vi "3458A Setup Virtual Channels.vi"(4 "LEVEL trigger":T1 caption="Cluster", 5 "sample period [s] (1 ms)":dbl=0.001 format="%#_6p", 6 "TRIG source (AUTO)":T2, 7 "apperture [s] (1.4 us)":dbl=1.4e-06 format="%#_6p", 8 "error in":errorcluster, 9 "samples count (100)":i32=100, 10 "voltage ranges [Vpk] (empty: use global default)":dbl[](array[numeric]), 11 "digitizer in":T3 {"channels"."Range [Vpk]" min=0.0}) -> (0 "error out":errorcluster, 3 "digitizer out":T3 {"channels"."Range [Vpk]" min=0.0})   [LabVIEW 2018, in "3458A Virtual Digitizer.lvlib"]
doc: "This VI setups all channels of a virtual digitizer to desired modes. If vector of ranges is entered it will override default channel settings from the session. It also setups all related instruments to the needed states (AWG and counter). Call this VI at least once before initiating digitizing!"
uses:
  3458A Virtual Digitizer.lvlib
  3458A Digitizer Session.ctl
  3458A Virtual Channel Config.ctl
  Counter/Counter Session.ctl
  Counter/Counter Type.ctl
  AWG/AWG Session.ctl
  AWG/AWG Type.ctl
  3458A Sync Mode.ctl
  3458A Idn Mode.ctl
  3458A Digitizing Low Levels/Configure/Sampling Mode.ctl
  3458A Digitizing Process Options.ctl
  3458A Data Packet.ctl
  3458A Aux Record Data.ctl
  3458A Digitizing Low Levels/Configure/Level Setup.ctl
  3458A Digitizing Low Levels/Configure/First Sample Trigger.ctl
  3458A Aperture Selection Mode.ctl
  3458A Digitizing Low Levels/Configure/EXT OUT mode.ctl
  <vilib>/Utility/error.llb/Error Cluster From Error Code.vi
  <vilib>/ErrorRing/Error Ring.xnode
  3458A Digitizing Low Levels/3458A Digitizing Low Levels.lvlib
  AWG/AWG.lvlib
  Counter/Counter.lvlib
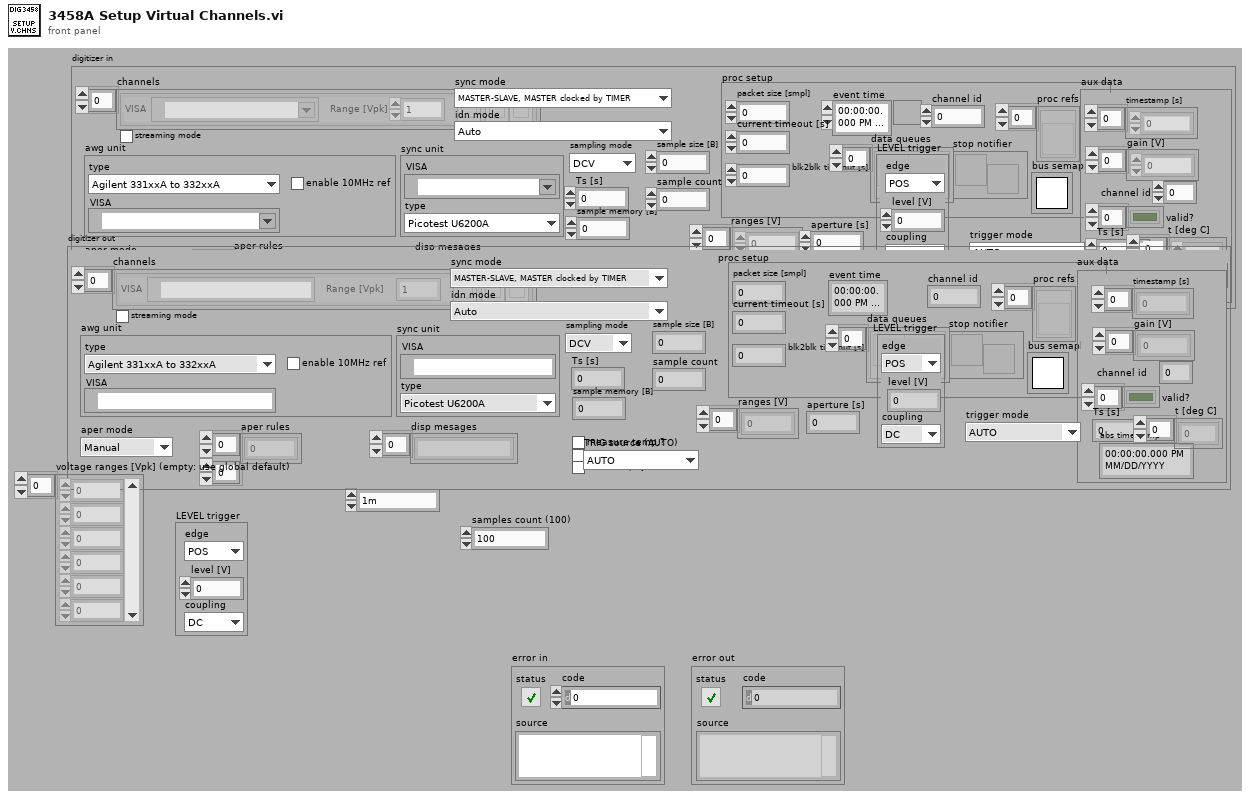
[diagram p1: front panel]
types:
  T1 = typedef "3458A Virtual Digitizer.lvlib/3458A Digitizing Low Levels.lvlib/Level Setup.ctl" = cluster{"edge":enum16{"POS", "NEG"}, "level [V]":dbl, "coupling":enum16{"DC", "AC"}}
  T2 = typedef "3458A Virtual Digitizer.lvlib/3458A Digitizing Low Levels.lvlib/First Sample Trigger.ctl" = enum16{"AUTO", "EXT", "SYN", "SGL", "HOLD", "LEVEL"}
  T3 = typedef "3458A Virtual Digitizer.lvlib/3458A Digitizer Session.ctl" = cluster{"channels":T4[], "sync unit":T5, "awg unit":T7, "sync mode":T9, "streaming mode":bool, "idn mode":T10, "sampling mode":T11, "Ts [s]":dbl, "sample memory [B]":i32, "proc setup":T12, "sample size [B]":i32, "sample count":i32, "aux data":T14, "ranges [V]":dbl[], "aperture [s]":dbl, "LEVEL trigger":T1, "trigger mode":T2, "measure temp.?":bool, "disp mesages":string[], "shared bus?":bool, "disable display?":bool, "aper mode":T15, "aper rules":dbl[][]}
  T4 = typedef "3458A Virtual Digitizer.lvlib/3458A Virtual Channel Config.ctl" = cluster{"VISA":refnum<visa-resource-name>, "Range [Vpk]":dbl, "btn clr":bool, "btn up":bool, "btn down":bool}
  T5 = typedef "Counter.lvlib/Counter Session.ctl" = cluster{"VISA":refnum<visa-resource-name>, "type":T6}
  T6 = typedef "Counter.lvlib/Counter Type.ctl" = enum16{"Picotest U6200A", "dummy"}
  T7 = typedef "AWG.lvlib/AWG Session.ctl" = cluster{"type":T8, "VISA":refnum<visa-resource-name>, "enable 10MHz ref":bool}
  T8 = typedef "AWG.lvlib/AWG Type.ctl" = enum16{"Agilent 331xxA to 332xxA", "Agilent 335xxA to 336xxA", "Tektronix AFG3101C", "dummy"}
  T9 = typedef "3458A Virtual Digitizer.lvlib/3458A Sync Mode.ctl" = enum16{"MASTER-SLAVE, MASTER clocked by TIMER", "MASTER-SLAVE, MASTER clocked by AWG", "ALL clocked by AWG", "MASTER-SLAVE, ALL clocked by TIMER", "ALL clocked by AWG with DFLL"}
  T10 = typedef "3458A Virtual Digitizer.lvlib/3458A Idn Mode.ctl" = enum16{"Auto", "Sequential (chn A, chn B, ...)", "From calibration string"}
  T11 = typedef "3458A Virtual Digitizer.lvlib/3458A Digitizing Low Levels.lvlib/Sampling Mode.ctl" = enum16{"DCV", "DSDC", "DSAC"}
  T12 = typedef "3458A Virtual Digitizer.lvlib/3458A Digitizing Process Options.ctl" = cluster{"channel id":i32, "packet size [smpl]":i32, "current timeout [s]":dbl, "blk2blk timeout [s]":dbl, "event time":timestamp, "stop notifier":refnum<notifier>, "data queues":refnum<queue>[], "proc refs":refnum<vi>[], "bus semaphore":T13}
  T13 = typedef "Semaphore RefNum" = refnum<k1>
  T14 = typedef "3458A Virtual Digitizer.lvlib/3458A Aux Record Data.ctl" = cluster{"channel id":i32, "valid?":bool[], "gain [V]":dbl[], "timestamp [s]":dbl[], "Ts [s]":dbl, "abs timestamp":timestamp, "t [deg C]":dbl[]}
  T15 = typedef "3458A Virtual Digitizer.lvlib/3458A Aperture Selection Mode.ctl" = enum16{"Manual", "Maximum", "Table"}
  T16 = typedef "3458A Virtual Digitizer.lvlib/3458A Digitizing Low Levels.lvlib/EXT OUT mode.ctl" = enum16{"APER", "ICOMP"}
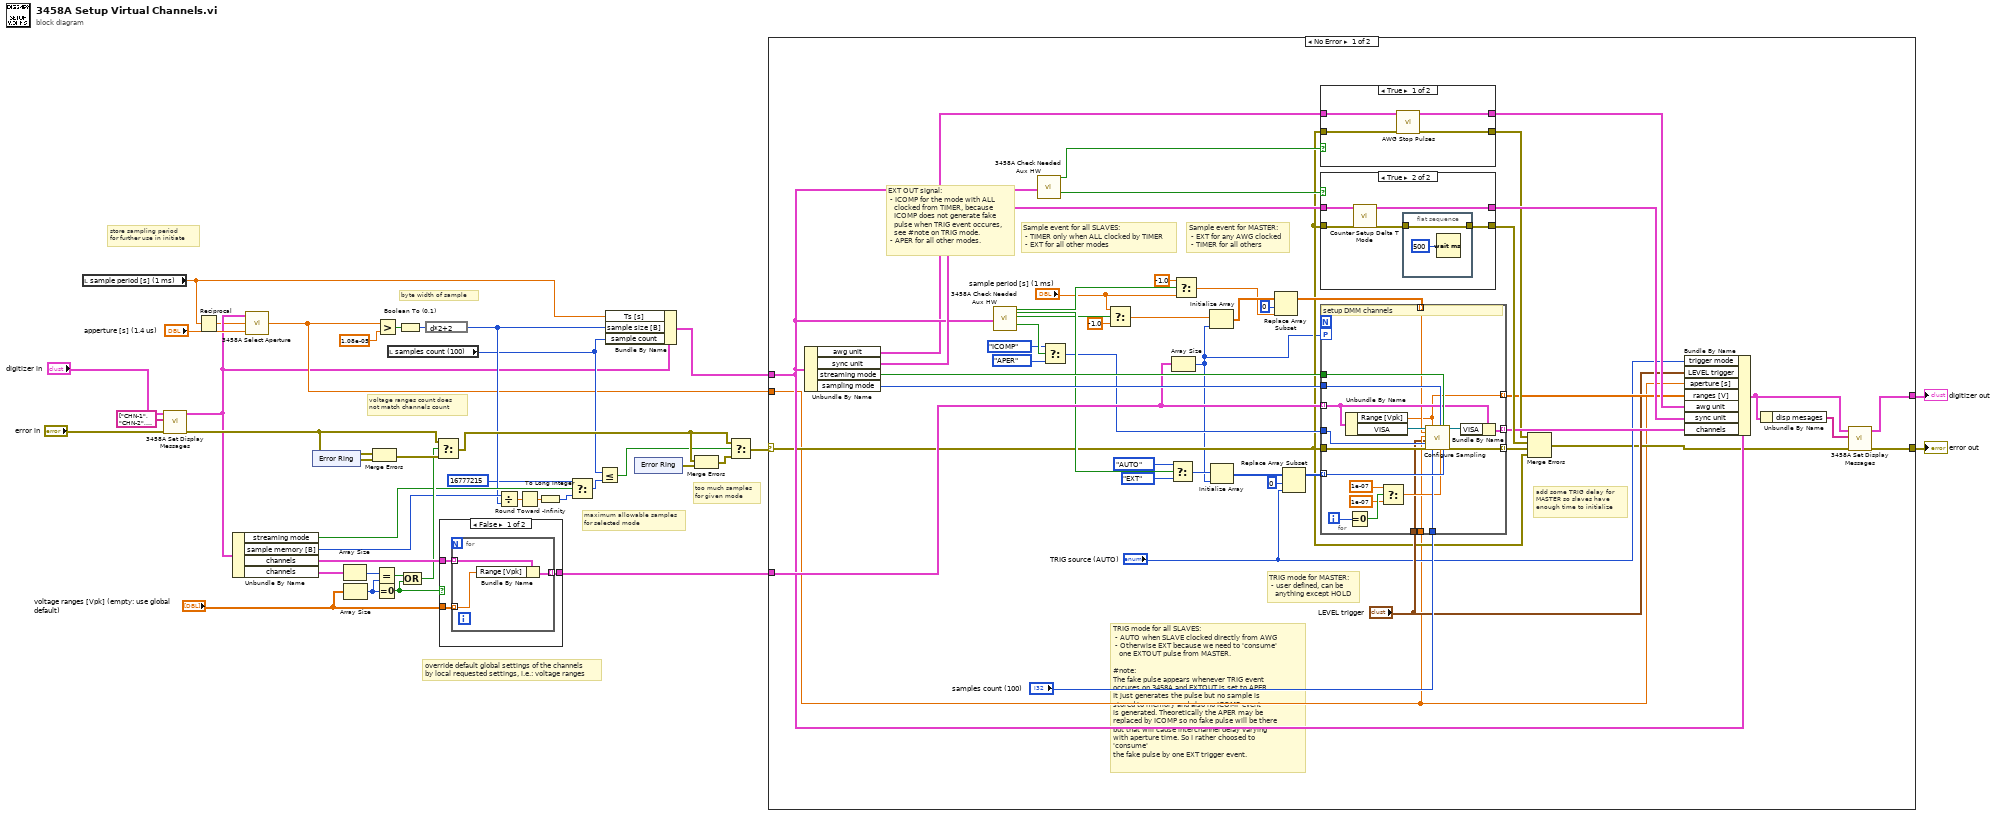
[diagram p0: block diagram]
diagram:
  # "store sampling period\nfor further use in initiate"
  # "voltage ranges count does\nnot match channels count"
  # "maximum allowable samples\nfor selected mode"
  # "byte width of sample"
  # "too much samples\nfor given mode"
  # "override default global settings of the channels\nby local requested settings, i.e.: voltage ranges"
  n1 = local read "sample period [s] (1 ms)"() -> (w2:dbl)
  n2 = call "3458A Set Display Messages.vi"("error in (no error)"="error in", "display strings"=string[] ["CHN-1", "CHN-2", "CHN-3"], "digitizer session in"="digitizer in") -> ("error out"=w8:errorcluster, "digitizer session out"=w3:T3)  [unwired: 7 in]
  n3 = Reciprocal(x=w2) -> (1/x=w1:dbl)
  n4 = Unbundle By Name(w3) -> ("streaming mode"=w21:bool, "sample memory [B]"=w16:i32, "channels"=w37:T4[], "channels"=w38:T4[])
  n5 = call "3458A Select Aperture.vi"("manual aperture [s]"="apperture [s] (1.4 us)", "sampling rate [Sa/s]"=w1, "digitizer session"=w3) -> ("selected aperture [s]"=w4:dbl)
  n6 = xnode "Error Ring"() -> ("error out"=w36:errorcluster)
  n7 = Array Size(array=w38) -> (size(s)=w26:i32)
  n8 = Array Size(array="voltage ranges [Vpk] (empty: use global default)") -> (size(s)=w30:i32)
  n9 = Merge Errors(w8, w36) -> (w35:errorcluster)
  n10 = Equal?(x=w26, y=w30) -> (x = y?=w31:bool)
  n11 = Equal To 0?(x=w30) -> (x = 0?=w27:bool)
  n12 = Greater?(x=w4, y=1.08e-05) -> (0:w24:bool)
  n13 = local read "samples count (100)"() -> (w12:i32)
  n14 = Boolean To (0,1)(Boolean=w24) -> (0, 1=w23:i16)
  n15 = Compound Arithmetic op=OR(w31, w27) -> (w29:bool)
  n16 = expression code="d*2+2"(w23) -> (w14:i16)
  n17 = Select(t=w8, s=w29, f=w35) -> (s? t:f=w32:errorcluster)
  n18 = case shown="False" w27 {
    tunnel: w37 -> [w43 w47]
    tunnel: [w42 w47] -> w17
    tunnel: "voltage ranges [Vpk] (empty: use global default)" -> [w41 _]
    frame False {
      n19 = for {
        tunnel: w43 -> [w46] mode=indexing
        tunnel: w41 -> [w44] mode=indexing
        tunnel: [w45] -> w42 mode=indexing
        n20 = Bundle By Name(cluster=w46, "Range [Vpk]"=w44) -> (w45:T4)
      }
    }
    frame True {
    }
  }
  n21 = Divide(x=w16, y=w14) -> (x/y=w15:dbl)
  n22 = Round Toward -Infinity(1:w15) -> (0:w11:dbl)
  n23 = To Long Integer(number=w11) -> (32bit integer=w10:i32)
  n24 = Select(t=16777215, s=w21, f=w10) -> (s? t:f=w22:i32)
  n25 = Less Or Equal?(x=w12, y=w22) -> (x <= y?=w20:bool)
  n26 = Bundle By Name(cluster=w3, "Ts [s]"=w2, "sample size [B]"=w14, "sample count"=w12) -> (w18:T3)
  n27 = xnode "Error Ring"() -> ("error out"=w33:errorcluster)
  n28 = Merge Errors(w32, w33) -> (w34:errorcluster)
  n29 = Select(t=w32, s=w20, f=w34) -> (s? t:f=w19:errorcluster)
  n30 = case shown="No Error" w19 {
    selector: w19 -> [w50 w131]
    tunnel: [w53 w130] -> w40
    tunnel: [w54 w131] -> w39
    tunnel: w18 -> [w72 w130]
    tunnel: w17 -> [w84 _]
    tunnel: w4 -> [w48 _]
    frame No Error {
      # "EXT OUT signal:\n - ICOMP for the mode with ALL\n   clocked from TIMER, because\n   ICOMP does not generate fake\n   pulse when TRIG event occures,\n   see #note on TRIG mode.\n - APER for all other modes."
      # "add some TRIG delay for\nMASTER so slaves have\nenough time to initialize"
      # "Sample event for MASTER:\n - EXT for any AWG clocked\n - TIMER for all others"
      # "Sample event for all SLAVES:\n - TIMER only when ALL clocked by TIMER\n - EXT for all other modes"
      # "TRIG mode for MASTER:\n - user defined, can be\n   anything except HOLD"
      # "TRIG mode for all SLAVES:\n - AUTO when SLAVE clocked directly from AWG\n - Otherwise EXT because we need to 'consume' \n   one EXTOUT pulse from MASTER.\n\n#note:\nThe fake pulse appears whenever TRIG event \noccures on 3458A and EXTOUT is set to APER.\nIt just generates the pulse but no sample is\nstored to memory and also no ICOMP event\nis generated. Theoretically the APER may be\nreplaced by ICOMP so no fake pulse will be there\nbut that will cause interchannel delay varying\nwith aperture time. So I rather choosed to 'consume'\nthe fake pulse by one EXT trigger event."
      n31 = Unbundle By Name(w72) -> ("awg unit"=w69:T7, "sync unit"=w90:T5, "streaming mode"=w88:bool, "sampling mode"=w87:T11)
      n32 = call "3458A Check Needed Aux HW.vi"("digitizer session"=w72) -> ("uses AWG clocking?"=w75:bool, "SLAVEs clocked by AWG?"=w73:bool, "SLAVEs clocked from TIMER?"=w66:bool, "uses counter for delta T sync?"=w63:bool)  [unwired: 13 in, 2 out]
      n33 = call "3458A Check Needed Aux HW.vi"("digitizer session"=w72) -> ("uses AWG clocking?"=w70:bool, "uses counter for delta T sync?"=w71:bool)  [unwired: 13 in, 4 out]
      n34 = Select(t=EXT_OUT_mode."ICOMP" ("EXT OUT signal (APER)"), s=w63, f=EXT_OUT_mode."APER" ("EXT OUT signal (APER)")) -> (s? t:f=w60:T16)
      n35 = Select(t="sample period [s] (1 ms)", s=w66, f=-1.0 ("t")) -> (s? t:f=w83:dbl)
      n36 = Select(t=First_Sample_Trigger."AUTO" ("first sample (AUTO)"), s=w73, f=First_Sample_Trigger."EXT" ("first sample (AUTO)")) -> (s? t:f=w77:T2)
      n37 = Array Size(array=w84) -> (size(s)=w49:i32)
      n38 = Select(t=-1.0, s=w75, f="sample period [s] (1 ms)") -> (s? t:f=w79:dbl)
      n39 = Initialize Array(w83, w49) -> (w82:dbl[])
      n40 = Initialize Array(w77, w49) -> (w93:T2[])
      n41 = Replace Array Subset(array=w82, new element=w79, index=0) -> (w80:dbl[])
      n42 = Replace Array Subset(array=w93, new element="TRIG source (AUTO)", index=0) -> (w91:T2[])
      n43 = case shown="True" w70 {
        tunnel: w50 -> [w98 w99]
        tunnel: [w96 w99] -> w68
        tunnel: w69 -> [w97 w100]
        tunnel: [w95 w100] -> w67
        frame True {
          # "init AWG for external sample clocking"
          n44 = call "AWG Stop Pulses.vi"("error in (no error)"=w98, "awg session in"=w97) -> ("error out"=w96:errorcluster, "awg session out"=w95:T7)  [unwired: 8 in]
        }
        frame False {
          # "init counter for two DMM delta T\nmeasurement"
        }
      }
      n45 = case shown="True" w71 {
        tunnel: w90 -> [w102 w104]
        tunnel: w50 -> [w101 w106]
        tunnel: [w101 w107] -> w89
        tunnel: [w102 w103] -> w85
        frame False {
        }
        frame True {
          # "init counter for two DMM delta T\nmeasurement"
          n46 = call "Counter Setup Delta T Mode.vi"("error in"=w106, "counter session in"=w104) -> ("error out"=w105:errorcluster, "counter session out"=w103:T5)  [unwired: 8 in]
          n47 = flat-sequence {
            tunnel: [w109] -> w107
            tunnel: w105 -> [w109]
            frame #0 {
              n48 = Wait (ms)(milliseconds to wait=u32 500) -> ()  [unwired: 1 out]
            }
          }
        }
      }
      n49 = for {
        tunnel: w50 -> [w129]
        tunnel: w84 -> [w122] mode=indexing
        tunnel: [w128] -> w94 mode=indexing
        tunnel: [w120] -> w86 mode=indexing
        tunnel: w48 -> [w112]
        tunnel: "samples count (100)" -> [w125]
        tunnel: w91 -> [w126] mode=indexing
        tunnel: w88 -> [w124]
        tunnel: w87 -> [w123]
        tunnel: w80 -> [w119] mode=indexing
        workers-P: w49 -> [_]
        tunnel: w60 -> [w113]
        tunnel: "LEVEL trigger" -> [w111]
        tunnel: [w110] -> w58 mode=indexing
        i -> [w118]
        # "setup DMM channels"
        n50 = Unbundle By Name(w122) -> ("Range [Vpk]"=w110:dbl, "VISA"=w127:refnum<visa-resource-name>)
        n51 = Equal To 0?(x=w118) -> (x = 0?=w117:bool)
        n52 = Select(t=1e-07, s=w117, f=1e-07) -> (s? t:f=w116:dbl)
        n53 = call "Configure Sampling.vi"("VISA resource in"=w127, "sample period [s] (-1: use EXT trig as source)"=w119, "apperture [s] (1.4us)"=w112, "LEVEL trigger"=w111, "EXT OUT signal (APER)"=w113, "error in"=w129, "range [V] (10V)"=w110, "samples count (100)"=w125, "sampling mode (DCV)"=w123, "delay [s]"=w116, "stream mode (False)"=w124, "first sample (AUTO)"=w126) -> ("VISA resource name out"=w121:refnum<visa-resource-name>, "error out"=w128:errorcluster)  [unwired: 6 in]
        n54 = Bundle By Name(cluster=w122, "VISA"=w121) -> (w120:T4)
      }
      n55 = Merge Errors(w68, w89, w94, w50) -> (w55:errorcluster)
      n56 = Bundle By Name(cluster=w72, "trigger mode"="TRIG source (AUTO)", "LEVEL trigger"="LEVEL trigger", "aperture [s]"=w48, "ranges [V]"=w58, "awg unit"=w67, "sync unit"=w85, "channels"=w86) -> (w52:T3)
      n57 = Unbundle By Name(w52) -> ("disp mesages"=w51:string[])
      n58 = call "3458A Set Display Messages.vi"("error in (no error)"=w55, "display strings"=w51, "digitizer session in"=w52) -> ("error out"=w54:errorcluster, "digitizer session out"=w53:T3)  [unwired: 7 in]
    }
    frame Error {
    }
  }
  "error out" <- w39
  "digitizer out" <- w40
